vi "InitSamplesData.vi"   [LabVIEW 2013]
uses:
  GlobalVariables/SamplesData.vi
types:
  T1 = cluster{"date":string, "sampleNumber":string, "sampleID":string, "sampleDepth":string, "dryWeight":string, "grainDensity":string, "bulkVolume":string, "poreVolume":string, "porosity":string, "sleeveVolume":string, "sleeveLength":string, "sleeveDiameter":string, "sleeveThickness":string, "temperature":string, "comments":string}[]
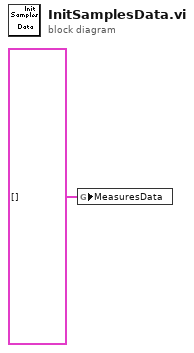
[diagram p0: block diagram]
diagram:
  n1 = global write "SamplesData.vi" "MeasuresData"(T1 [] ("MeasuresData")) -> ()
